vi "ini_read_cplx_extended_vector.vi"(7 "section":string, 8 "error in":errorcluster, 9 "default":cxt[](array[numeric]), 10 "key":string, 11 "refnum in":T1) -> (0 "error out":errorcluster, 1 "values":cxt[](array[numeric]), 2 "found?":bool, 3 "refnum out":T1)   [LabVIEW 2013]
uses:
  <vilib>/Utility/config.llb/Config Data RefNum.ctl
  <vilib>/Utility/config.llb/Read Key (String).vi
  <vilib>/Utility/config.llb/NI_LVConfig.lvlib
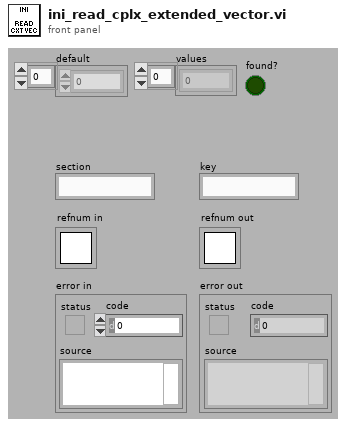
[diagram p1: front panel]
types:
  T1 = typedef "NI_LVConfig.lvlib/Config Data RefNum.ctl" = refnum<k1>
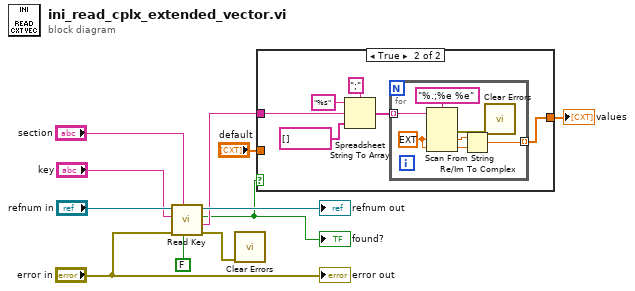
[diagram p0: block diagram]
diagram:
  n1 = call-poly <vilib>:"Read Key.vi"("read raw string? (F)"=FALSE, "section"="section", "error in (no error)"="error in", "key"="key", "refnum"="refnum in") -> ("error out"=w6:errorcluster, "value"=w5:string, "found?"=w4:bool, "refnum out"=→"refnum out":T1)  [unwired: 3 in]
  "found?" <- w4
  n2 = call <vilib>:"Clear Errors.vi"("error in (no error)"=w6) -> ()  [unwired: 6 in, 1 out]
  n3 = case shown="True" w4 {
    tunnel: w5 -> [_ w14]
    tunnel: "default" -> [w12 _]
    tunnel: [w12 w13] -> w2
    frame False {
    }
    frame True {
      n4 = Spreadsheet String To Array(delimiter (Tab)=";", format string="%s", spreadsheet string=w14, array type (2D Dbl)=string[] []) -> (array=w16:string[])
      n5 = for {
        tunnel: w16 -> [w25] mode=indexing
        tunnel: [w21] -> w13 mode=indexing
        w19 = ext 0.0 ("default value 1")
        n6 = Scan From String(format string="%.;%e %e", input string=w25, default 1=w19, default 2=w19) -> (error out=w20:errorcluster, output 1=w23:ext, output 2=w22:ext)  [unwired: 2 in, 2 out]
        n7 = Re/Im To Complex(1:w22, 2:w23) -> (0:w21:cxt)
        n8 = call <vilib>:"Clear Errors.vi"("error in (no error)"=w20) -> ()  [unwired: 6 in, 1 out]
      }
    }
  }
  "values" <- w2
  "error out" <- "error in"
